vi "VIE.Module.Queued Message Handler.enqueue.State.QueuedMessageHandler.vi"   [LabVIEW 2010, in "VIE.Module.Queued Message Handler.QueuedMessageHandler.dqGOOPClass.lvlib"]
uses:
  VIE.Module.Queued Message Handler.QueuedMessageHandler.dqGOOPClass.lvlib
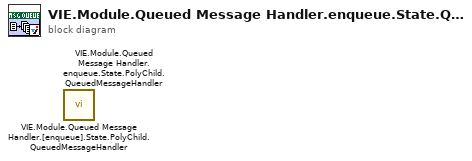
[diagram p0: block diagram]
diagram:
  n1 = call "VIE.Module.Queued Message Handler.[enqueue].State.PolyChild.QueuedMessageHandler.vi"() -> ()  [unwired: 10 in, 2 out]
  n2 = call "VIE.Module.Queued Message Handler.enqueue.State.PolyChild.QueuedMessageHandler.vi"() -> ()  [unwired: 10 in, 2 out]
